vi "Write Play.vi"(6 "Current Selected Play":T1, 7 "Commit Play Changes":bool, 9 "filename array":string[](array[string]), 10 "Is a File":bool, 11 "File Refnum":refnum<vi>) -> (2 "File Write Error":errorcluster, 3 "Not Cancelled\nLoad File":bool)   [LabVIEW 2015]
uses:
  Autonomous VIs/Autonomous Exec/Autonomous Play Definition.ctl
  Autonomous VIs/Autonomous Commands/Autonomous Command Names.ctl
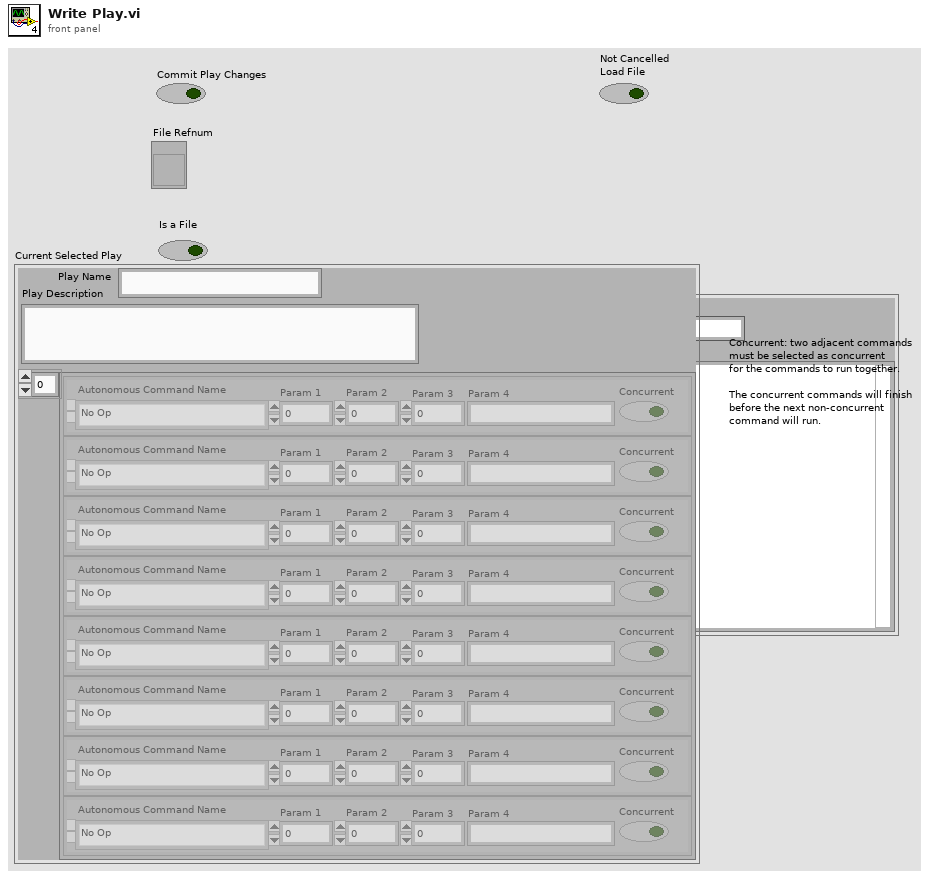
[diagram p1: front panel]
types:
  T1 = typedef "Autonomous Play Definition.ctl" = cluster{"Play Name":string, "Command List":cluster{"Param 1":dbl, "Param 2":dbl, "Autonomous Command Name":T2, "Concurrent":bool, "Param 3":dbl, "Param 4":string}[], "Play Description":string}
  T2 = typedef "Autonomous Command Names.ctl" = enum16{"No Op", "Drive Time", "Run Motion Profile", "Turn to Heading", "Turn To Target", "Cross Defense", "Fire", "Wait", "Reset Gyro", "Grabber Setpoints", "Manual Grabber", "Roller", "Autorange Command", "Reposition"}
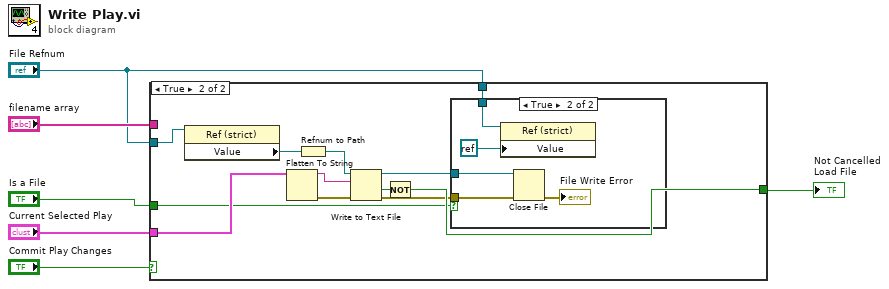
[diagram p0: block diagram]
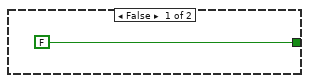
[diagram p2: hidden frame]
diagram:
  n1 = case shown="True" "Commit Play Changes" {
    tunnel: [FALSE w18] -> w3
    tunnel: "Current Selected Play" -> [_ w16]
    tunnel: "filename array" -> [_ _]
    tunnel: "File Refnum" -> [_ w11]
    tunnel: "Is a File" -> [_ w9]
    tunnel: "File Refnum" -> [_ w10]
    frame False {
    }
    frame True {
      n2 = property class="Ref (strict)"(reference=w11) -> ("Value"=w13:refnum<file>)  [unwired: 1 in, 2 out]
      n3 = Flatten To String(anything=w16) -> (data string=w8:string, error out=w15:errorcluster)  [unwired: 3 in, 1 out]
      n4 = Refnum to Path(1:w13) -> (0:w12:path)
      n5 = Write to Text File(file (use dialog)=w12, text=w8, error in=w15) -> (refnum out=w17:refnum<file>, cancelled=w19:bool, error out=w14:errorcluster)  [unwired: 1 in]
      n6 = Not(x=w19) -> (.not. x?=w18:bool)
      n7 = case shown="True" w9 {
        tunnel: w17 -> [_ w24]
        tunnel: w14 -> [_ w20]
        tunnel: w10 -> [_ w21]
        frame False {
        }
        frame True {
          n8 = property class="Ref (strict)"(reference=w21, "Value"=refnum<k0> refnum) -> ()  [unwired: 1 in, 2 out]
          n9 = Close File(refnum=w24, error in=w20) -> (error out=→"File Write Error":errorcluster)  [unwired: 1 out]
        }
      }
    }
  }
  "Not Cancelled\nLoad File" <- w3
